vi "DeleteSeqStruct.vi"(9 "Multiframe Stuct in":refnum<vi>) -> ()   [LabVIEW 2021, in "MemberVICreation.lvlib" / "BaseAccessorScripter.lvclass"]
uses:
  <resource>/Framework/Providers/LVClassLibrary/NewAccessors/BaseAccessorScripter/BaseAccessorScripter.lvclass
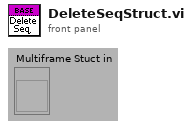
[diagram p1: front panel]
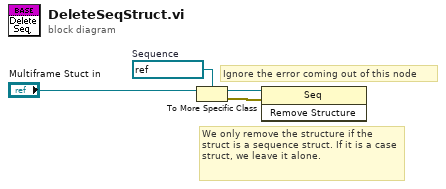
[diagram p0: block diagram]
diagram:
  w3 = refnum<vi> refnum  # Sequence
  # "We only remove the structure if the struct is a sequence struct. If it is a case struct, we leave it alone."
  # "Ignore the error coming out of this node"
  n1 = To More Specific Class(target class=w3, reference="Multiframe Stuct in") -> (specific class reference=w1:refnum<vi>, error out=w2:errorcluster)  [unwired: 1 in]
  n2 = invoke class="Seq" method="Remove Structure"(reference=w1, error in=w2) -> ()  [unwired: 1 in, 3 out]
